vi "SENS_OFFS_STAT.vi"(0 "VISA IN":refnum<visa-resource-name>, 1 "Frq. Offset ON/OFF":bool, 5 "error in":errorcluster, 7 "Channel":i32) -> (14 "VISA Out":refnum<visa-resource-name>, 19 "error out":errorcluster)   [LabVIEW 2018, in "PNA-X.lvlib"]
doc: "SENSe<cnum>:OFFSet:[STATe] <bool> \n(Read-Write) Enables Frequency Offset Mode on ALL measurements that are present on the active \nchannel. This immediately causes the source and receiver to tune to separate frequencies. The receiver \nfrequencies are specified with the other SENS:OFFSet commands. To make the stimulus settings use \nthe SENS:FREQ commands. \nTip: To avoid unnecessary errors, first make other offset frequency settings, then set Frequency Offset \nON. \nParameters \n<cnum> Any existing channel number. If unspecified, value is set to 1 \n<bool> ON (or 1) - turns Frequency Offset ON. \nOFF (or 0) - turns Frequency Offset OFF. \n1792\n\nExamples SENS:OFFS ON \nsense2:offset:state off \nQuery Syntax SENSe<cnum>:OFFSet:[STATe]? \nReturn Type Boolean \nDefault OFF (0)"
uses:
  PNA-X.lvlib
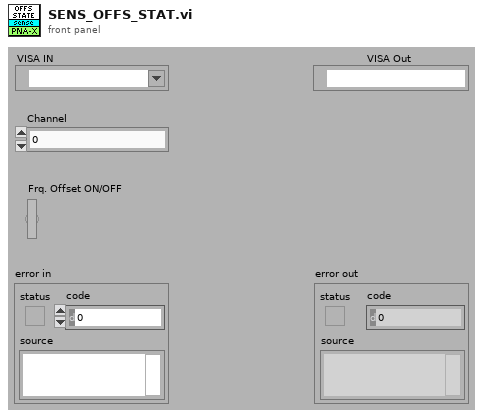
[diagram p1: front panel]
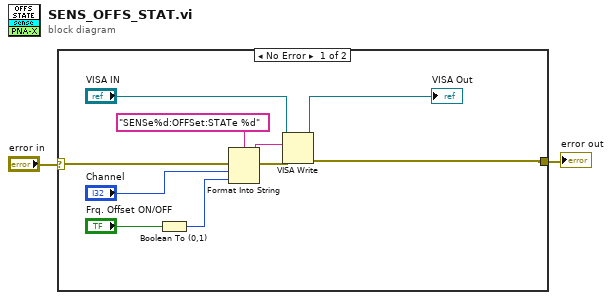
[diagram p0: block diagram]
diagram:
  n1 = case shown="No Error" "error in" {
    selector: "error in" -> [w12 w13]
    tunnel: [w7 w13] -> w1
    frame No Error {
      n2 = Boolean To (0,1)(Boolean="Frq. Offset ON/OFF") -> (0, 1=w3:i16)
      n3 = Format Into String(format string="SENSe%d:OFFSet:STATe %d" ("Cmdline"), error in=w12, "Channel", w3) -> (resulting string=w10:string, error out=w11:errorcluster)  [unwired: 1 in]
      n4 = VISA Write(VISA resource name="VISA IN", write buffer=w10, error in (no error)=w11) -> (VISA resource name out=→"VISA Out":refnum<visa-resource-name>, error out=w7:errorcluster)  [unwired: 1 out]
    }
    frame Error {
    }
  }
  "error out" <- w1
